vi "Target Fnc & Deriv NonLin2.vi"(2 "X":dbl format="%.3f", 3 "Coefficients":dbl[](array[numeric]) format="%.5f", 4 "Flag":enum16{"no deriv", "deriv"}(ring)) -> (0 "Derivatives":dbl[](array[numeric]) format="%.5f", 1 "Y":dbl format="%.3f")   [LabVIEW 2009]
doc: "Here the user specifies his guess at the functional form of the relationship between Y and X as a function of coefficients. \n\nIf the partial derivatives of the function are known, the user also furnishes the equations for the partial derivatives of this function with respect to each coefficient. The input control Flag should then be set to 1 (deriv) by all calling VIs.\n\nIf the partial derivatives of the function are not known, the input control Flag should be set to 0 (no deriv) by all calling VIs, and a numerical approximation to the partial derivatives will be computed."
panel:
  # "This VI calculates the output Y as a function of the input array X as well as the derivatives of the function at all values of X. The user specifies the \"Target Function\" and its derivatives in the formula nodes of this VI. The function describes the relationship of Y to X and the coefficients used are updated in each iteration after a new guess at their value is taken. Hence Y, Derivatives, and Coefficients are continuously changing."
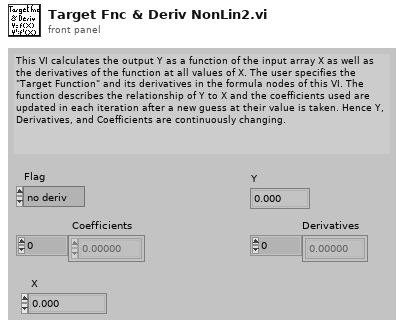
[diagram p1: front panel]
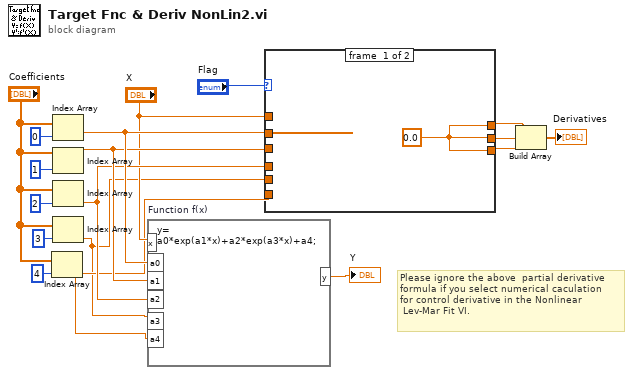
[diagram p0: block diagram]
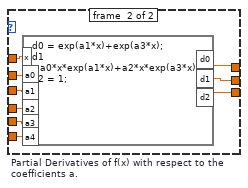
[diagram p2: hidden frame]
diagram:
  # "Please ignore the above  partial derivative \nformula if you select numerical caculation \nfor control derivative in the Nonlinear\n Lev-Mar Fit VI."
  n1 = Index Array(array="Coefficients", index=4) -> (element=w4:dbl)
  n2 = Index Array(array="Coefficients", index=0) -> (element=w14:dbl)
  n3 = Index Array(array="Coefficients", index=1) -> (element=w13:dbl)
  n4 = Index Array(array="Coefficients", index=2) -> (element=w12:dbl)
  n5 = Index Array(array="Coefficients", index=3) -> (element=w3:dbl)
  n6 = formula code="y= a0*exp(a1*x)+a2*exp(a3*x)+a4;" "Function f(x)"("x"="X", "a0"=w14, "a1"=w13, "a2"=w12, "a3"=w3, "a4"=w4) -> ("y"=→"Y":dbl)
  n7 = case shown="\"deriv\".." "Flag" {
    tunnel: "X" -> [_ w22]
    tunnel: [w19 w23] -> w9
    tunnel: [w19 w24] -> w10
    tunnel: [w19 w25] -> w11
    tunnel: w12 -> [_ w26]
    tunnel: w13 -> [_ w27]
    tunnel: w14 -> [_ w28]
    tunnel: w3 -> [_ w21]
    tunnel: w4 -> [_ w20]
    frame #0 {
      w19 = 0.0
    }
    frame #1 {
      n8 = formula code="d0 = exp(a1*x)+exp(a3*x);\nd1 =a0*x*exp(a1*x)+a2*x*exp(a3*x);\nd2 = 1;" "Partial Derivatives of f(x) with respect to the coefficients a."("x"=w22, "a0"=w28, "a1"=w27, "a2"=w26, "a3"=w21, "a4"=w20) -> ("d0"=w25:dbl, "d1"=w24:dbl, "d2"=w23:dbl)
    }
  }
  n9 = Build Array(w11, w10, w9) -> (→"Derivatives":dbl[])
